vi "numberrecognise2.vi"() -> ()   [LabVIEW 2019]
uses:
  <vilib>/userDefined/High Color/IMAQdx.ctl
  <vilib>/vision/driver/NI_Vision_Acquisition_Software.lvlib
panel:
  out "Image":T1(plugin-control)
  in  "stop":bool
  out "Image 2":T1(plugin-control)
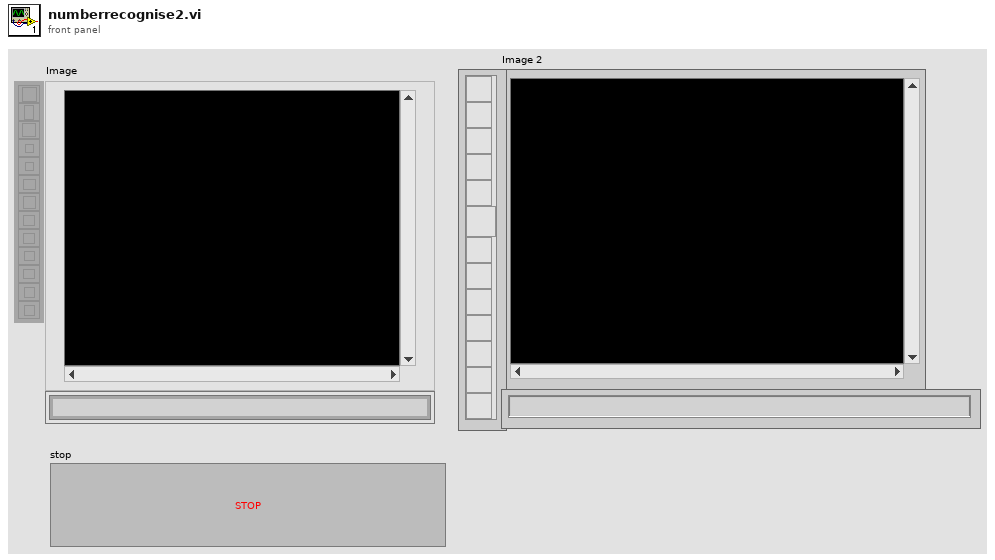
[diagram p1: front panel]
types:
  T1 = typedef "IMAQ Image.ctl" = refnum<image>
  T2 = typedef "IMAQdx.ctl" = refnum<k21>
  T3 = typedef "IMAQ Rectangle" = cluster{"Left":i32, "Top":i32, "Right":i32, "Bottom":i32, "Rotation":dbl}
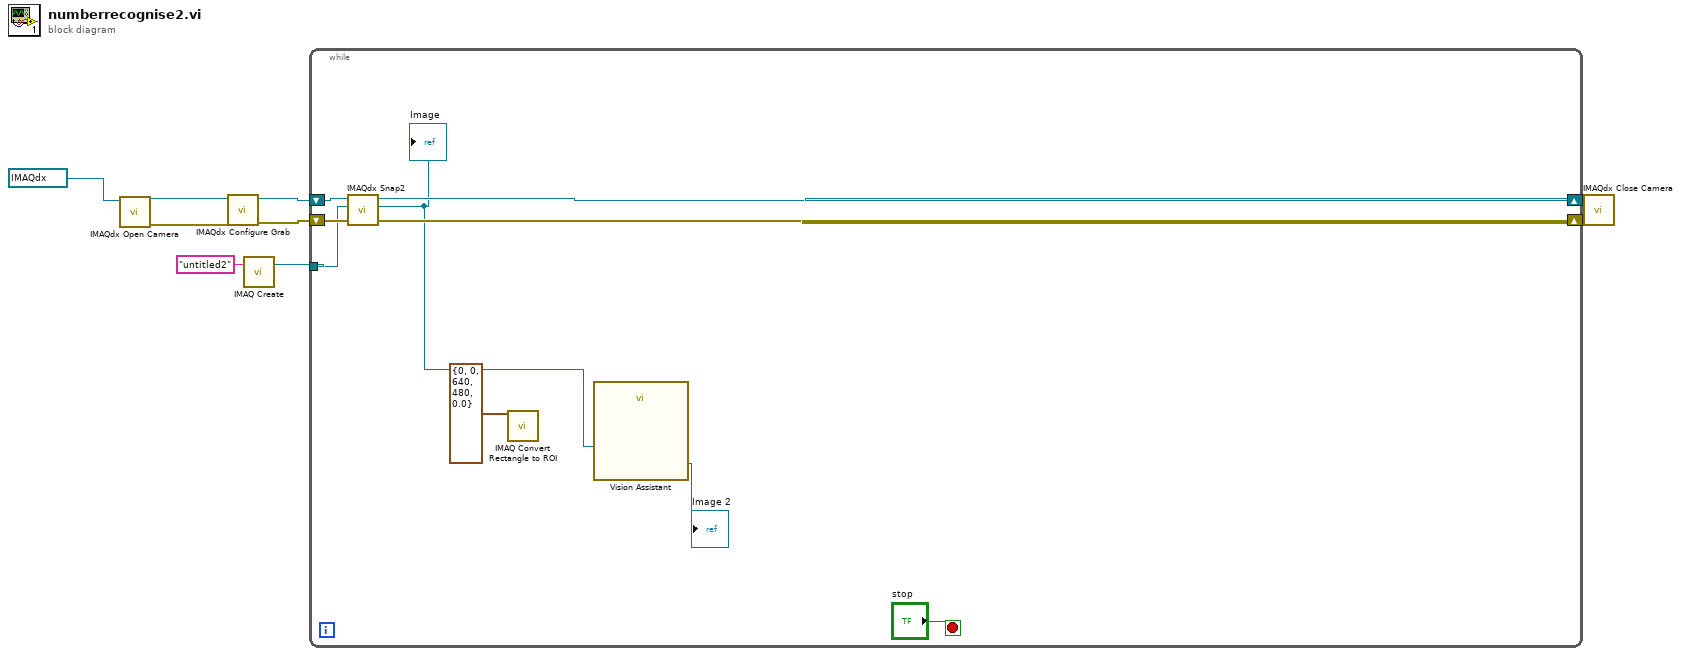
[diagram p0: block diagram]
diagram:
  n1 = call <vilib>:"IMAQdx Open Camera.vi"("Session In"=T2 "cam5") -> ("error out"=w5:errorcluster, "Session Out"=w8:T2)  [unwired: 9 in]
  n2 = call <vilib>:"IMAQdx Configure Grab.vi"("error in"=w5, "Session In"=w8) -> ("error out"=w4:errorcluster, "Session Out"=w7:T2)  [unwired: 8 in]
  n3 = call "IMAQ Create"("Image Name"="untitled2") -> ("New Image"=w1:T1)  [unwired: 4 in, 1 out]
  n4 = while {
    tunnel: w1 -> [w12]
    shift-right: [w17] -> w6
    shift-left: w7 -> [w18]
    shift-right: [w15] -> w3
    shift-left: w4 -> [w16]
    stop <- "stop" stop-if-true
    n5 = call <vilib>:"IMAQdx Snap2.vi"("error in"=w16, "Image In"=w12, "Session In"=w18) -> ("error out"=w15:errorcluster, "Image Out"=w11:T1, "Session Out"=w17:T2)  [unwired: 6 in]
    "Image" <- w11
    n6 = call "IMAQ Convert Rectangle to ROI"("Rectangle"=T3 {"Left"=0, "Top"=0, "Right"=640, "Bottom"=480, "Rotation"=0.0}) -> ()  [unwired: 8 in, 2 out]
    n7 = call "Vision Assistant"("Image In"=w11) -> ("Image Out"=→"Image 2":T1)  [unwired: 25 in, 1 out]
  }
  n8 = call <vilib>:"IMAQdx Close Camera.vi"("error in"=w3, "Session In"=w6) -> ()  [unwired: 9 in, 1 out]
